vi "GetComputerId.vi"(4 "error in (no error)":errorcluster) -> (0 "error out":errorcluster, 3 "ComuterId":string)   [LabVIEW 2011]
panel:
  out "Command Line:":string
  # "This VI just a command-line wrapper call to \"GetComputerId.exe\""
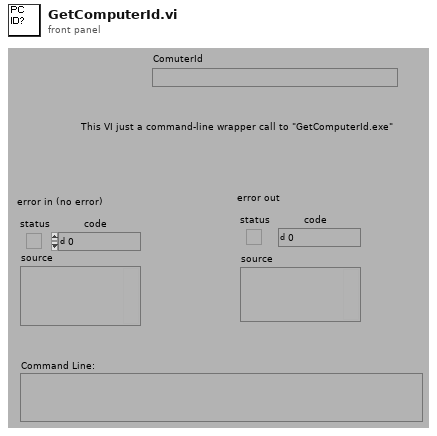
[diagram p1: front panel]
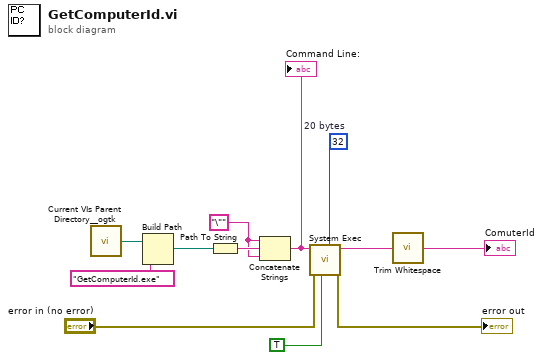
[diagram p0: block diagram]
diagram:
  w3 = u32 32  # 20 bytes
  w6 = "\""
  n1 = call <userlib>:"Current VIs Parent Directory__ogtk.vi"() -> ("Parent Directory (+ Relative)"=w10:path)  [unwired: 5 out]
  n2 = Build Path(base path=w10, name or relative path="GetComputerId.exe") -> (appended path=w8:path)
  n3 = Path To String(path=w8) -> (string=w7:string)
  n4 = Concatenate Strings(w6, w7, w6) -> (w5:string)
  "Command Line:" <- w5
  n5 = call <vilib>:"System Exec.vi"("expected output size  (4096)"=w3, "run minimized? (F)"=TRUE, "error in (no error)"="error in (no error)", "command line"=w5) -> ("error out"=→"error out":errorcluster, "standard output"=w2:string)  [unwired: 3 in, 3 out]
  n6 = call <vilib>:"Trim Whitespace.vi"("string"=w2) -> ("trimmed string"=→"ComuterId":string)  [unwired: 1 in]
